vi "Class Children Data.vi"(7 "Destination":path=path "", 8 "Error In":errorcluster, 11 "Class In":refnum<vi>) -> (0 "Error Out":errorcluster, 2 "Array":refnum<class "Map.lvclass">[](array[class]), 3 "Class Out":refnum<vi>)   [LabVIEW 2018, in "Scripts.lvlib"]
uses:
  Scripts.lvlib
  Toolkit/Data/Map/Map.lvclass
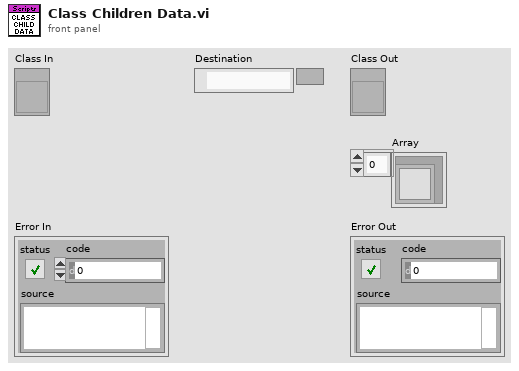
[diagram p1: front panel]
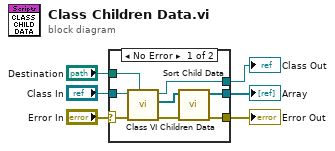
[diagram p0: block diagram]
diagram:
  n1 = case shown="No Error" "Error In" {
    selector: "Error In" -> [w9 w16]
    tunnel: [w13 _] -> w6
    tunnel: [w14 w16] -> w5
    tunnel: "Class In" -> [w12 w15]
    tunnel: "Destination" -> [w10 _]
    tunnel: [w11 w15] -> w1
    frame No Error {
      n2 = call "Class VI Children Data.vi"("Destination"=w10, "Error In"=w9, "Class In"=w12) -> ("Error Out"=w8:errorcluster, "Data"=w7:refnum<class "Map.lvclass">[], "Class Out"=w11:refnum<vi>)  [unwired: 6 in]
      n3 = call "Sort Child Data.vi"("Error In"=w8, "Unsorted In"=w7) -> ("Error Out"=w14:errorcluster, "Sorted Out"=w13:refnum<class "Map.lvclass">[])  [unwired: 8 in]
    }
    frame Error {
    }
  }
  "Array" <- w6
  "Error Out" <- w5
  "Class Out" <- w1
